vi "Dictionary Filter by Excluded.vi"(10 "Words_Ref in":refnum<vi>[](array[refnum]), 11 "Dictionary in":string[](array[string])) -> (3 "Dictionary out":string[](array[string]))   [LabVIEW 2015]
uses:
  TypeDef/Color.ctl
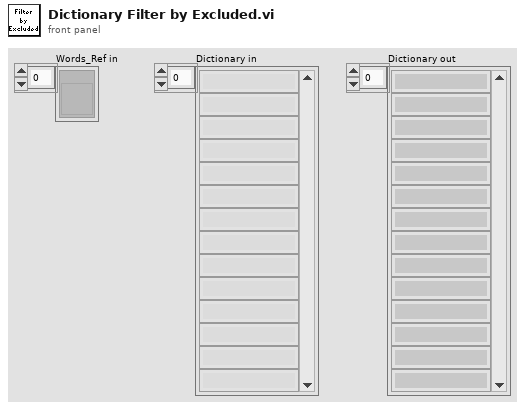
[diagram p1: front panel]
types:
  T1 = typedef "Color.ctl" = u32
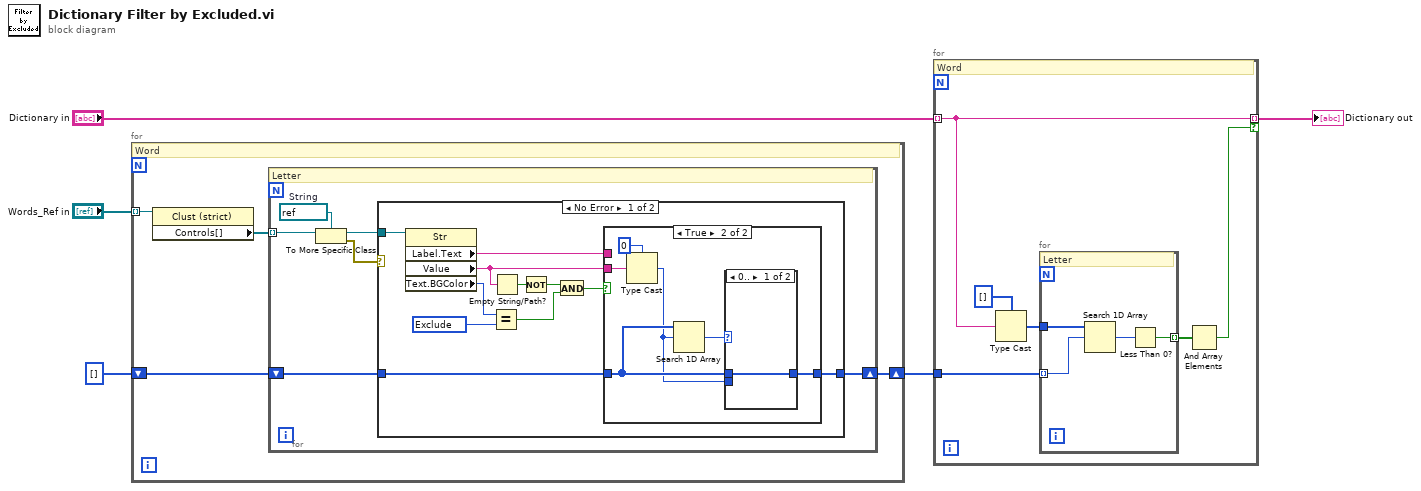
[diagram p0: block diagram]
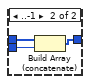
[diagram p3: hidden frame]
diagram:
  n1 = for {
    tunnel: "Words_Ref in" -> [w8] mode=indexing
    shift-right: [w6] -> w3
    shift-left: u8[] [] -> [w7]
    # "Word"
    n2 = property class="Clust (strict)"(reference=w8) -> ("Controls[]"=w9:refnum<vi>[])  [unwired: 1 in, 2 out]
    n3 = for {
      tunnel: w9 -> [w13] mode=indexing
      shift-right: [w14] -> w6
      shift-left: w7 -> [w15]
      w11 = refnum<vi> refnum  # String
      # "Letter"
      n4 = To More Specific Class(target class=w11, reference=w13) -> (specific class reference=w12:refnum<vi>, error out=w10:errorcluster)  [unwired: 1 in]
      n5 = case shown="No Error" w10 {
        tunnel: w15 -> [w25 w38]
        tunnel: [w24 w38] -> w14
        tunnel: w12 -> [w23 _]
        frame No Error {
          w20 = T1 12369084 items=["Free"=9567230, "Letter"=16774186, "Any"=16448250, "Exclude"=12369084] ("Color")
          n6 = property class="Str"(reference=w23) -> ("Label.Text"=w26:string, "Value"=w16:string, "Text.BGColor"=w21:u32)  [unwired: 1 in, 2 out]
          n7 = Equal?(x=w21, y=w20) -> (x = y?=w18:bool)
          n8 = Empty String/Path?(string/path=w16) -> (empty?=w22:bool)
          n9 = Not(x=w22) -> (.not. x?=w19:bool)
          n10 = And(x=w19, y=w18) -> (x .and. y?=w17:bool)
          n11 = case shown="True" w17 {
            tunnel: w26 -> [_ _]
            tunnel: w25 -> [w27 w30]
            tunnel: [w27 w33] -> w24
            tunnel: w16 -> [_ w31]
            frame False {
            }
            frame True {
              n12 = Type Cast(type=u8 0, x=w31) -> (*(type *) &x=w28:u8)
              n13 = Search 1D Array(1D array=w30, element=w28) -> (index of element=w29:i32)  [unwired: 1 in]
              n14 = case shown="0.." w29 {
                tunnel: [w34 w37] -> w33
                tunnel: w30 -> [w34 w36]
                tunnel: w28 -> [_ w35]
                frame 0.. {
                }
                frame ..-1 {
                  n15 = Build Array (concatenate)(w36, w35) -> (w37:u8[])
                }
              }
            }
          }
        }
        frame Error {
        }
      }
    }
  }
  n16 = for {
    tunnel: w3 -> [w44]
    tunnel: "Dictionary in" -> [w41] mode=indexing
    tunnel: [w41] -> w1 mode=indexing if=w39
    # "Word"
    n17 = Type Cast(type=u8[] [], x=w41) -> (*(type *) &x=w43:u8[])
    n18 = for {
      tunnel: w44 -> [w47] mode=indexing
      tunnel: w43 -> [w48]
      tunnel: [w45] -> w40 mode=indexing
      # "Letter"
      n19 = Search 1D Array(1D array=w48, element=w47) -> (index of element=w46:i32)  [unwired: 1 in]
      n20 = Less Than 0?(x=w46) -> (x < 0?=w45:bool)
    }
    n21 = And Array Elements(Boolean array=w40) -> (logical AND=w39:bool)
  }
  "Dictionary out" <- w1
